vi "Receive Messages.vi"(8 "Error In":errorcluster, 10 "Sender":string, 11 "Communicator in":refnum<class "Communicator.lvclass">) -> (0 "Error Out":errorcluster, 2 "Messages":refnum<class "IMessage.lvclass">[](array[class]), 3 "Communicator out":refnum<class "Communicator.lvclass">)   [LabVIEW 2019, in "Communicator.lvclass"]
uses:
  Communicator.lvclass
  Interfaces/IMessage/IMessage.lvclass
  Communicator Worker/Communicator Worker Messages/Receive Messages Msg/Get Messages Msg.lvclass
  <vilib>/ActorFramework/Specialty Messages/Reply Msg/Reply Msg.lvclass
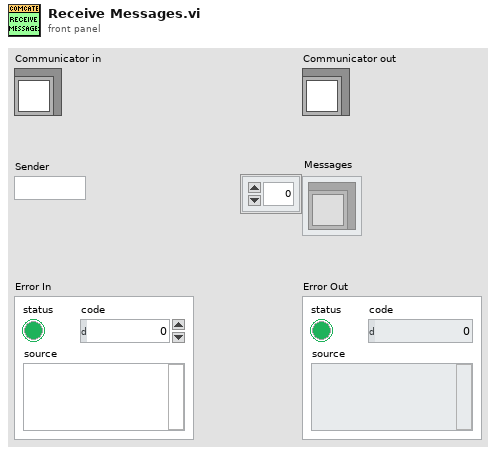
[diagram p1: front panel]
types:
  T1 = typedef "Communicator.lvclass/ObjectAttributes.ctl" = cluster{"IConfigure":refnum<class "IConfigure.lvclass">, "Worker Enqueuer":refnum<class "Message Enqueuer.lvclass">, "Start Counter":i32, "Msg Sent":refnum<user-event>}
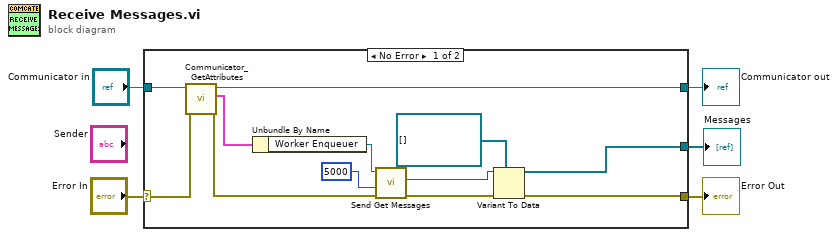
[diagram p0: block diagram]
diagram:
  n1 = case shown="No Error" "Error In" {
    selector: "Error In" -> [w16 w19]
    tunnel: [w13 w19] -> w4
    tunnel: [w15 w18] -> w2
    tunnel: "Communicator in" -> [w17 w18]
    tunnel: [w12 _] -> w1
    frame No Error {
      n2 = call "Communicator_GetAttributes.vi"("Error In"=w16, "Communicator in"=w17) -> ("Error Out"=w14:errorcluster, "Data"=w6:T1, "Communicator out"=w15:refnum<class "Communicator.lvclass">)  [unwired: 6 in, 1 out]
      n3 = Unbundle By Name(w6) -> ("Worker Enqueuer"=w11:refnum<class "Message Enqueuer.lvclass">)
      n4 = call "Send Get Messages.vi"("error in (no error)"=w14, "timeout in ms (-1)"=5000, "Message Enqueuer"=w11) -> ("error out"=w10:errorcluster, "Reply"=w7:variant)  [unwired: 5 in, 2 out]
      n5 = Variant To Data(error in=w10, type=refnum<class "IMessage.lvclass">[] [], Variant=w7) -> (data=w12:refnum<class "IMessage.lvclass">[], error out=w13:errorcluster)
    }
    frame Error {
    }
  }
  "Error Out" <- w4
  "Communicator out" <- w2
  "Messages" <- w1
